vi "Bin 2D Array 8 bit.vi"(1 "Input Array":u16[][](array[numeric]), 2 "Binning Value":u16) -> (0 "Binned Array":u8[][](array[numeric]))   [LabVIEW 2013]
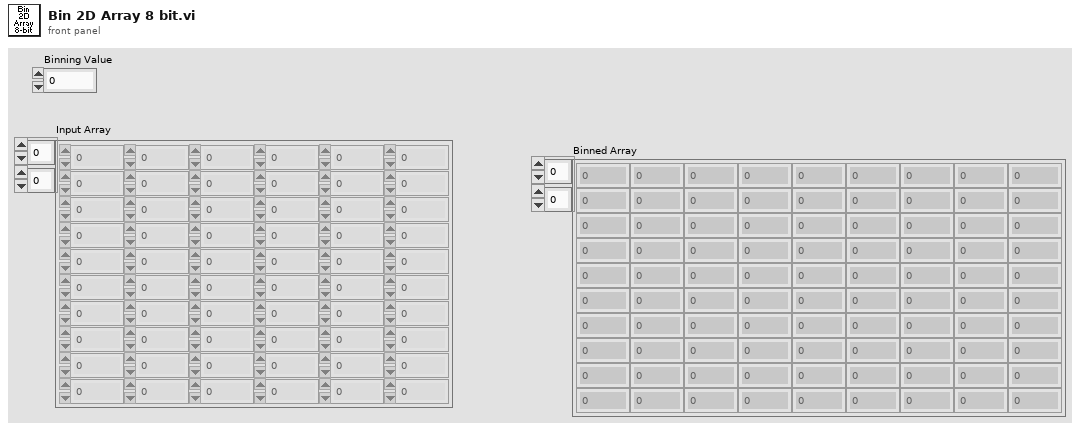
[diagram p1: front panel]
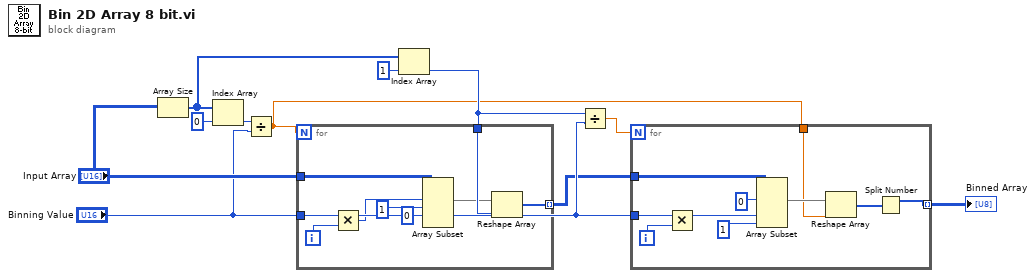
[diagram p0: block diagram]
diagram:
  n1 = Array Size(array="Input Array") -> (size(s)=w7:i32[])
  n2 = Index Array(array=w7, index=0) -> (element=w9:i32)
  n3 = Divide(x=w9, y="Binning Value") -> (x/y=w4:dbl)
  n4 = Index Array(array=w7, index=1) -> (element=w6:i32)
  n5 = for {
    N: w4 -> [_]
    tunnel: "Input Array" -> [w18]
    tunnel: "Binning Value" -> [w19]
    tunnel: [w17] -> w2 mode=indexing
    tunnel: w6 -> [w16]
    i -> [w20]
    n6 = Multiply(x=w19, y=w20) -> (x*y=w14:i32)
    n7 = Array Subset(array=w18, index (row)=w14, length (row)=1 ("length"), index (col)=0 ("index")) -> (w15:u16[][])  [unwired: 1 in]
    n8 = Reshape Array(w15, w16) -> (w17:u16[])
  }
  n9 = Divide(x=w6, y="Binning Value") -> (x/y=w5:dbl)
  n10 = for {
    N: w5 -> [_]
    tunnel: w2 -> [w28]
    tunnel: "Binning Value" -> [w29]
    tunnel: [w21] -> w1 mode=indexing
    tunnel: w4 -> [w23]
    i -> [w30]
    n11 = Multiply(x=w29, y=w30) -> (x*y=w25:i32)
    n12 = Array Subset(array=w28, index (row)=0 ("index"), index (col)=w25, length (col)=1 ("length")) -> (w27:u16[][])  [unwired: 1 in]
    n13 = Reshape Array(w27, w23) -> (w22:u16[])
    n14 = Split Number(x=w22) -> (hi(x)=w21:u8[])  [unwired: 1 out]
  }
  "Binned Array" <- w1
